vi "programa9.vi"() -> ()   [LabVIEW 2011]
panel:
  in  "On/Off Prg":bool
  out "Temperatura Minima":dbl
  out "Temperatura Maxima":dbl
  out "Temperatura Promedio":dbl
  in  "On/Off A/C":bool
  out "A/C On":bool
  in  "Temperatura Deseada":dbl
  out "Temperatura":i32(slide) scale=0.0..50.0
  # "El programa simula el funcionamiento de un a/c \ndonde se ingresa la temperatura deseada y cada vez\nque la temperatura deseada sea mayor a temperatura \nno se enciende el a/c , pero cuando esta sea menor se\nenciende el compresor pero esto solo puede ocurrir\nsiempre el a/c este encendido, el programa termina solo \ncuando decidimos nosotros terminar."
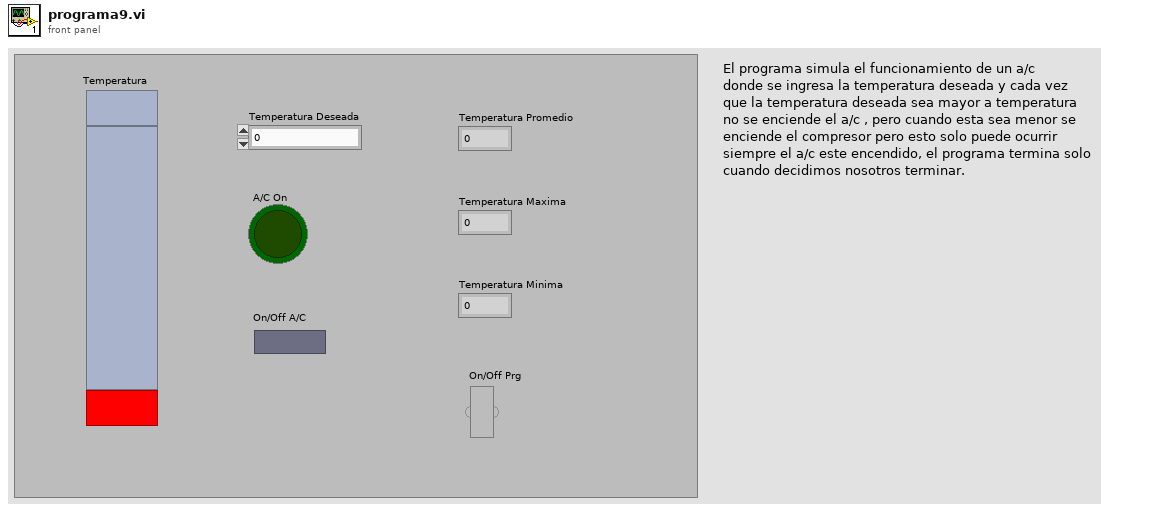
[diagram p1: front panel]
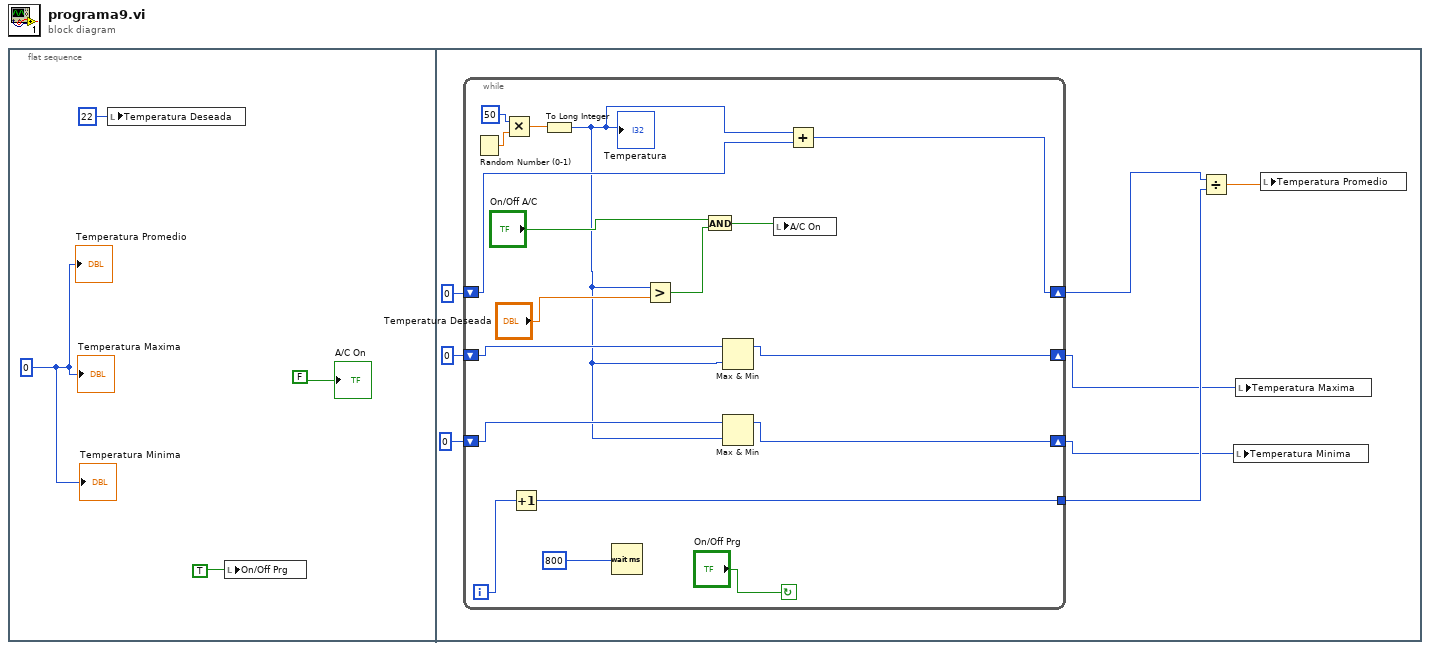
[diagram p0: block diagram]
diagram:
  n1 = flat-sequence {
    frame #0 {
      w4 = 0
      n2 = local write "Temperatura Deseada"(22) -> ()
      n3 = local write "On/Off Prg"(TRUE) -> ()
      "A/C On" <- FALSE
      "Temperatura Promedio" <- w4
      "Temperatura Maxima" <- w4
      "Temperatura Minima" <- w4
    }
    frame #1 {
      n4 = while {
        tunnel: [w21] -> w11
        shift-right: [w18] -> w9
        shift-left: 0 -> [w19]
        shift-right: [w14] -> w6
        shift-left: 0 -> [w17]
        shift-right: [w13] -> w5
        shift-left: 0 -> [w16]
        i -> [w22]
        stop <- "On/Off Prg" continue-if-true
        n5 = Random Number (0-1)() -> (number: 0 to 1=w29:dbl)
        n6 = Multiply(x=50, y=w29) -> (x*y=w27:dbl)
        n7 = Increment(x=w22) -> (x+1=w21:i32)
        n8 = To Long Integer(number=w27) -> (32bit integer=w15:i32)
        "Temperatura" <- w15
        n9 = Wait (ms)(milliseconds to wait=800) -> ()  [unwired: 1 out]
        n10 = Greater?(x=w15, y="Temperatura Deseada") -> (0:w25:bool)
        n11 = And(x="On/Off A/C", y=w25) -> (x .and. y?=w23:bool)
        n12 = Max & Min(x=w17, y=w15) -> (max(x,y)=w14:i32)  [unwired: 1 out]
        n13 = Max & Min(x=w16, y=w15) -> (max(x,y)=w13:i32)  [unwired: 1 out]
        n14 = local write "A/C On"(w23) -> ()
        n15 = Add(x=w15, y=w19) -> (x+y=w18:i32)
      }
      n16 = Divide(x=w9, y=w11) -> (x/y=w12:dbl)
      n17 = local write "Temperatura Minima"(w5) -> ()
      n18 = local write "Temperatura Maxima"(w6) -> ()
      n19 = local write "Temperatura Promedio"(w12) -> ()
    }
  }
